vi "Event Loop Wrapper.vi"(10 "Actor":refnum<class "Actor.lvclass">, 11 "Panel in":refnum<class "Helper Loop.lvclass">) -> ()   [LabVIEW 2021, in "Helper Loop.lvclass"]
uses:
  Helper Loop.lvclass
  <vilib>/jettl/jettl/Actor/Actor/Actor.lvclass
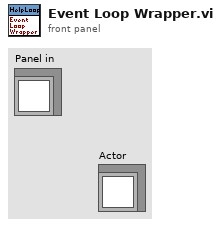
[diagram p1: front panel]
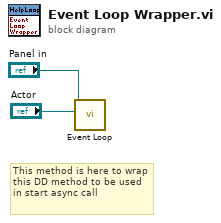
[diagram p0: block diagram]
diagram:
  # "This method is here to wrap this DD method to be used in start async call"
  n1 = call-dynamic "Event Loop.vi"("Actor"="Actor", "Panel"="Panel in") -> ()  [unwired: 10 in]
